vi "dfd_Get Alternate Components of Array.vi"   [LabVIEW 2017, in "NI_DigFilterLicensed.lvlib"]
uses:
  <vilib>/addons/Digital Filter Design/NI_DigFilterLicensed.lvlib
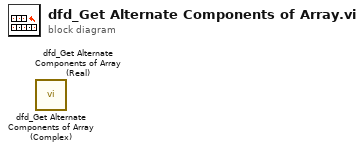
[diagram p0: block diagram]
diagram:
  n1 = call <vilib>:"dfd_Get Alternate Components of Array (Complex).vi"() -> ()  [unwired: 10 in, 2 out]
  n2 = call <vilib>:"dfd_Get Alternate Components of Array (Real).vi"() -> ()  [unwired: 10 in, 2 out]
